vi "LS218_READ_TYPE_SONDES.vi"(0 "Refnum VISA en entrée":refnum<visa-resource-name>, 1 "Voies A ou B":string, 2 "entrée d'erreur (pas d'erreur)":errorcluster) -> (3 "Nom de ressource VISA en sortie":refnum<visa-resource-name>, 5 "Input_type":i32, 6 "sortie d'erreur":errorcluster)   [LabVIEW 2016]
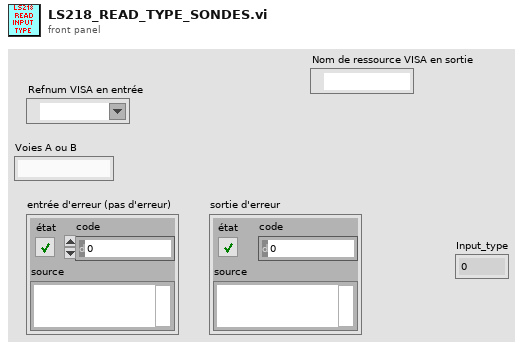
[diagram p1: front panel]
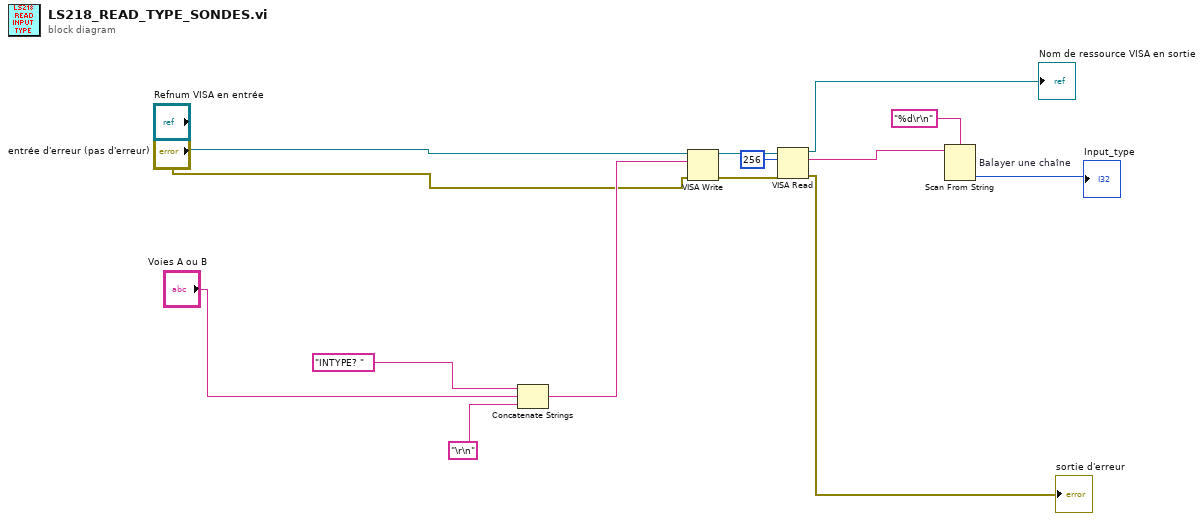
[diagram p0: block diagram]
diagram:
  n1 = Concatenate Strings("INTYPE? " ("chaîne"), "Voies A ou B", "\r\n" ("chaîne")) -> (w7:string)
  n2 = VISA Write(VISA resource name="Refnum VISA en entrée", write buffer=w7, error in (no error)="entrée d'erreur (pas d'erreur)") -> (VISA resource name out=w14:refnum<visa-resource-name>, error out=w13:errorcluster)  [unwired: 1 out]
  n3 = VISA Read(VISA resource name=w14, byte count=u32 256 ("nombre d'octets"), error in (no error)=w13) -> (VISA resource name out=→"Nom de ressource VISA en sortie":refnum<visa-resource-name>, read buffer=w5:string, error out=→"sortie d'erreur":errorcluster)  [unwired: 1 out]
  n4 = Scan From String "Balayer une chaîne"(format string="%d\r\n" ("chaîne de format"), input string=w5) -> (output 1=→"Input_type":i32)  [unwired: 3 in, 3 out]
